vi "set_buffer_arrays.vi"(8 "error in (no error)":errorcluster, 10 "Buffer arrays":refnum<data-value>[](array[refnum]), 11 "ImageAssemblerRK110612Spiral in":refnum<class "ImageAssemblerRK110612Spiral.lvclass">) -> (0 "error out":errorcluster, 3 "ImageAssemblerRK110612Spiral out":refnum<class "ImageAssemblerRK110612Spiral.lvclass">)   [LabVIEW 2010, in "ImageAssemblerRK110612Spiral.lvclass"]
uses:
  ImageAssemblerRK110612Spiral.lvclass
  ImageAssemblerRK110612Spiral.lvclass/ImageAssemblerRK110612Spiral.ctl
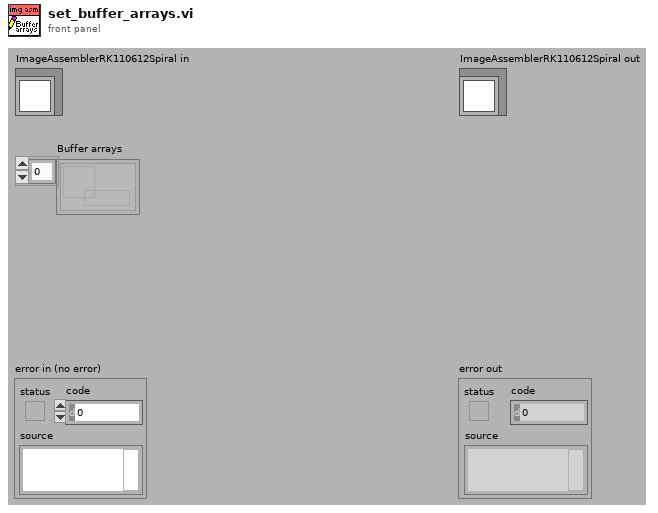
[diagram p1: front panel]
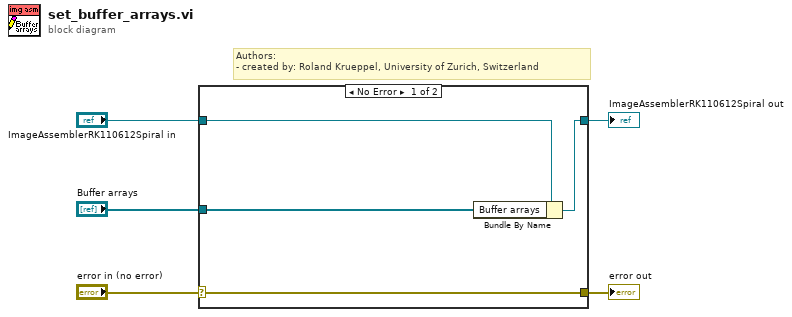
[diagram p0: block diagram]
diagram:
  # "Authors: \n- created by: Roland Krueppel, University of Zurich, Switzerland"
  n1 = case shown="No Error" "error in (no error)" {
    selector: "error in (no error)" -> [w9 w10]
    tunnel: [w9 w10] -> w4
    tunnel: [w7 w11] -> w2
    tunnel: "ImageAssemblerRK110612Spiral in" -> [w8 w11]
    tunnel: "Buffer arrays" -> [w6 _]
    frame No Error {
      n2 = Bundle By Name(cluster=w8, "Buffer arrays"=w6) -> (w7:refnum<class "ImageAssemblerRK110612Spiral.lvclass">)
    }
    frame Error {
    }
  }
  "error out" <- w4
  "ImageAssemblerRK110612Spiral out" <- w2
